vi "1st Derivative of Rational Polynomial (DBL).vi"(9 "GCD?":bool=TRUE, 10 "Q(x)":dbl[](array[numeric]) min=0.0 max=127.0 format="%#.6g", 11 "P(x)":dbl[](array[numeric]) min=0.0 max=127.0 format="%#.6g") -> (0 "error":i32, 2 "Denominator d[P(x)/Q(x)]/dx":dbl[](array[numeric]), 3 "Numerator d[P(x)/Q(x)]/dx":dbl[](array[numeric]))   [LabVIEW 2014, in "NI_AALPro.lvlib"]
uses:
  NI_AALPro.lvlib
  nth Derivative of Polynomial (DBL).vi
  Multiply Polynomials (DBL).vi
  Subtract Polynomials (DBL).vi
  GCD of P(x) and Q(x) (DBL).vi
  Divide Polynomials (DBL).vi
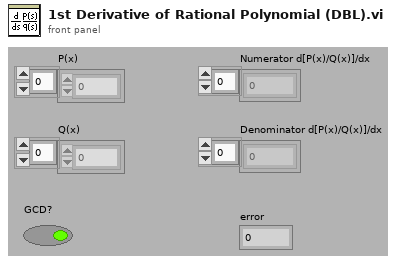
[diagram p1: front panel]
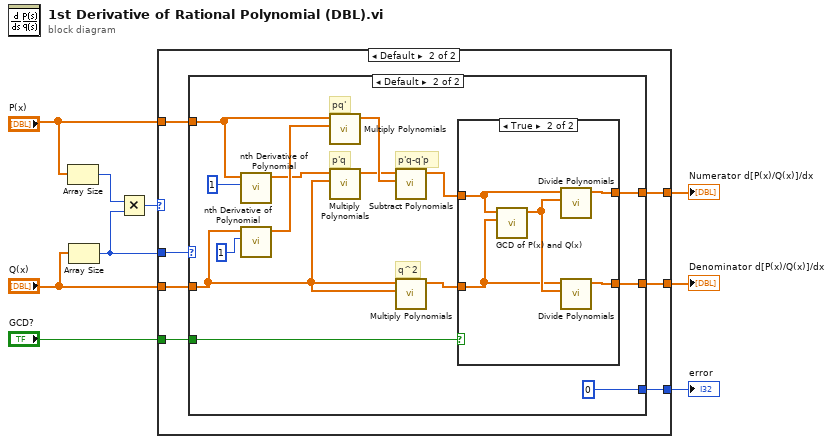
[diagram p0: block diagram]
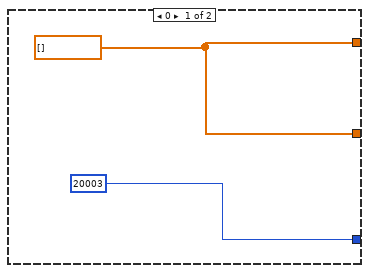
[diagram p2: hidden frame]
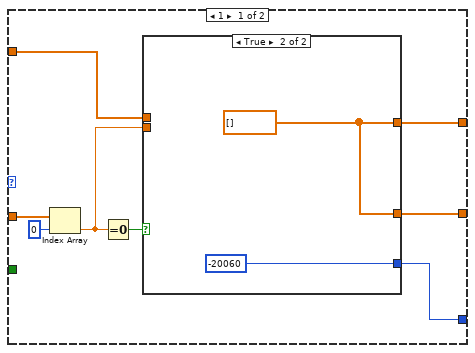
[diagram p3: hidden frame]
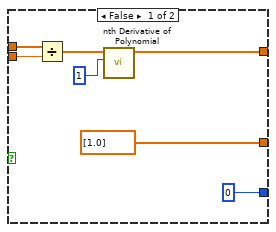
[diagram p4: hidden frame]
diagram:
  n1 = Array Size(array="P(x)") -> (size(s)=w4:i32)
  n2 = Array Size(array="Q(x)") -> (size(s)=w3:i32)
  n3 = Multiply(x=w4, y=w3) -> (x*y=w2:i32)
  n4 = case shown="Default" w2 {
    tunnel: "P(x)" -> [_ w18]
    tunnel: [w11 w17] -> w9
    tunnel: [w11 w16] -> w8
    tunnel: "Q(x)" -> [_ w15]
    tunnel: [20003 ("empty array") w13] -> w5
    tunnel: w3 -> [_ w14]
    tunnel: "GCD?" -> [_ w12]
    frame 0 {
      w11 = dbl[] []
    }
    frame Default {
      n5 = case shown="Default" w14 {
        tunnel: w18 -> [w20 w47]
        tunnel: [w23 w46] -> w17
        tunnel: [w22 w41] -> w16
        tunnel: w15 -> [w26 w40]
        tunnel: [w21 0] -> w13
        tunnel: w12 -> [_ w36]
        frame 1 {
          n6 = Index Array(array=w26, index=0) -> (element=w19:dbl)
          n7 = Equal To 0?(x=w19) -> (x = 0?=w24:bool)
          n8 = case shown="True" w24 {
            tunnel: [w30 w35] -> w23
            tunnel: [dbl[] [1.0] w35] -> w22
            tunnel: [0 ("divide by zero") -20060 ("divide by zero")] -> w21
            tunnel: w20 -> [w33 _]
            tunnel: w19 -> [w32 _]
            frame False {
              n9 = Divide(x=w33, y=w32) -> (x/y=w31:dbl[])
              n10 = call-poly "nth Derivative of Polynomial.vi"("order"=1, "P(x)"=w31) -> ("Nth Derivative of P(x)"=w30:dbl[])  [unwired: 8 in, 1 out]
            }
            frame True {
              w35 = dbl[] []
            }
          }
        }
        frame Default {
          # "q^2"
          # "p'q"
          # "pq'"
          # "p'q-q'p"
          n11 = call-poly "nth Derivative of Polynomial.vi"("order"=1, "P(x)"=w47) -> ("Nth Derivative of P(x)"=w44:dbl[])  [unwired: 8 in, 1 out]
          n12 = call-poly "nth Derivative of Polynomial.vi"("order"=1, "P(x)"=w40) -> ("Nth Derivative of P(x)"=w45:dbl[])  [unwired: 8 in, 1 out]
          n13 = call-poly "Multiply Polynomials.vi"("Q(x)"=w45, "P(x)"=w47) -> ("P(x)*Q(x)"=w49:dbl[])  [unwired: 8 in, 1 out]
          n14 = call-poly "Multiply Polynomials.vi"("Q(x)"=w40, "P(x)"=w44) -> ("P(x)*Q(x)"=w43:dbl[])  [unwired: 8 in, 1 out]
          n15 = call-poly "Subtract Polynomials.vi"("Q(x)"=w49, "P(x)"=w43) -> ("P(x)-Q(x)"=w48:dbl[])  [unwired: 8 in, 1 out]
          n16 = call-poly "Multiply Polynomials.vi"("Q(x)"=w40, "P(x)"=w40) -> ("P(x)*Q(x)"=w42:dbl[])  [unwired: 8 in, 1 out]
          n17 = case shown="True" w36 {
            tunnel: w48 -> [w51 w53]
            tunnel: [w51 w56] -> w46
            tunnel: w42 -> [w50 w52]
            tunnel: [w50 w54] -> w41
            frame False {
            }
            frame True {
              n18 = call-poly "GCD of P(x) and Q(x).vi"("Q(x)"=w52, "P(x)"=w53) -> ("Greatest Common Divisor"=w55:dbl[])  [unwired: 8 in, 1 out]
              n19 = call-poly "Divide Polynomials.vi"("Q(x)"=w55, "P(x)"=w53) -> ("P(x)/Q(x)"=w56:dbl[])  [unwired: 7 in, 2 out]
              n20 = call-poly "Divide Polynomials.vi"("Q(x)"=w55, "P(x)"=w52) -> ("P(x)/Q(x)"=w54:dbl[])  [unwired: 7 in, 2 out]
            }
          }
        }
      }
    }
  }
  "Numerator d[P(x)/Q(x)]/dx" <- w9
  "Denominator d[P(x)/Q(x)]/dx" <- w8
  "error" <- w5
